vi "test Get and Set TX Start Time.vi"(8 "error in (no error)":errorcluster, 11 "TestCase in":refnum<class "Framework Status Tests.lvclass">) -> (0 "error out":errorcluster, 3 "TestCase out":refnum<class "Framework Status Tests.lvclass">)   [LabVIEW 2017, in "Framework Status Tests.lvclass"]
uses:
  Framework Status Tests.lvclass
  Engine/Classes/Status/Framework Performance.lvclass/Framework Performance.ctl
  <vilib>/addons/_JKI Toolkits/VI Tester/TestCase.llb/TestCase.lvclass
  Engine/Classes/Status/Framework Performance.lvclass
  C:/Program Files (x86)/National Instruments/LabVIEW 2017/vi.lib/addons/_JKI Toolkits/VI Tester/TestCase.llb/TestCase.lvclass
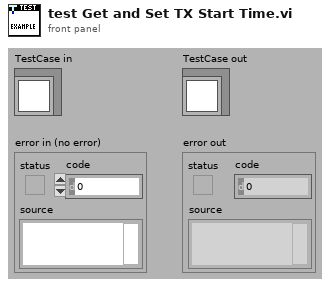
[diagram p1: front panel]
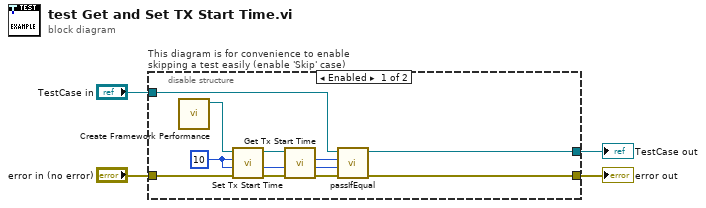
[diagram p0: block diagram]
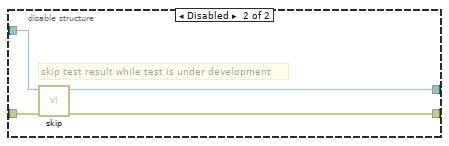
[diagram p2: hidden frame]
diagram:
  n1 = disable-structure "This diagram is for convenience to enable skipping a test easily (enable 'Skip' case)" shown="Enabled" {
    disable-tunnel: "TestCase in" -> [w8 w16]
    disable-tunnel: [w7 w14] -> w1
    disable-tunnel: [w9 w15] -> w3
    disable-tunnel: "error in (no error)" -> [w12 w13]
    frame Enabled {
      w5 = u32 10 ("Tx start time")
      n2 = call "Create Framework Performance.vi"() -> ("Framework Performance"=w11:refnum<class "Framework Performance.lvclass">)  [unwired: 10 in, 1 out]
      n3 = call "Set Tx Start Time.vi"("Tx start time"=w5, "Framework Performance in"=w11) -> ("Framework Performance out"=w10:refnum<class "Framework Performance.lvclass">)  [unwired: 9 in]
      n4 = call "Get Tx Start Time.vi"("Framework Performance in"=w10) -> ("Tx start time"=w6:u32)  [unwired: 9 in, 1 out]
      n5 = call-dynamic "passIfEqual.vi"("error in (no error)"=w12, "y"=w5, "x"=w6, "TestCase in"=w8) -> ("error out"=w9:errorcluster, "TestCase out"=w7:refnum<class "Framework Status Tests.lvclass">)  [unwired: 6 in]
    }
    frame Disabled {
      # "skip test result while test is under development"
      n6 = call <vilib>:"skip.vi"("error in (no error)"=w13, "TestCase in"=w16) -> ("error out"=w15:errorcluster, "TestCase out"=w14:refnum<class "Framework Status Tests.lvclass">)  [unwired: 8 in]
    }
  }
  "error out" <- w3
  "TestCase out" <- w1
